vi "BMP180 Pull Raw Measurement.vi"(6 "Sensor Type":enum16{"Temp", "Pressure"}(ring), 8 "error in (no error)":errorcluster, 9 "BMP180 Config":T7={"I2C"={"Slave Address"=64, "Channel"=0}, "Mode"=enum."Ultra Low Power", "Cal Coefs"={"AC1"={"Addr:"=0, "Val:"=0}, "AC2"={"Addr:"=0, "Val:"=0}, "AC3"={"Addr:"=0, "Val:"=0}, "AC4"={"Addr:"=0, "Val:"=0}, "AC5"={"Addr:"=0, "Val:"=0}, "AC6"={"Addr:"=0, "Val:"=0}, "B1"={"Addr:"=0, "Val:"=0}, "B2"={"Addr:"=0, "Val:"=0}, "MB"={"Addr:"=0, "Val:"=0}, "MC"={"Addr:"=0, "Val:"=0}, "MD"={"Addr:"=0, "Val:"=0}}} {"I2C"."Slave Address" format="%.0x"; "Cal Coefs"."MD"."Val:" format="%04x"; "Cal Coefs"."MD"."Addr:" format="%02x"; "Cal Coefs"."MC"."Val:" format="%04x"; "Cal Coefs"."MC"."Addr:" format="%02x"; "Cal Coefs"."MB"."Val:" format="%04x"; "Cal Coefs"."MB"."Addr:" format="%02x"; "Cal Coefs"."B2"."Val:" format="%04x"; "Cal Coefs"."B2"."Addr:" format="%02x"; "Cal Coefs"."B1"."Val:" format="%04x"; "Cal Coefs"."B1"."Addr:" format="%02x"; "Cal Coefs"."AC6"."Val:" format="%04x"; "Cal Coefs"."AC6"."Addr:" format="%02x"; "Cal Coefs"."AC5"."Val:" format="%04x"; "Cal Coefs"."AC5"."Addr:" format="%02x"; "Cal Coefs"."AC4"."Val:" format="%04x"; "Cal Coefs"."AC4"."Addr:" format="%02x"; "Cal Coefs"."AC3"."Val:" format="%04x"; "Cal Coefs"."AC3"."Addr:" format="%02x"; "Cal Coefs"."AC2"."Val:" format="%04x"; "Cal Coefs"."AC2"."Addr:" format="%02x"; "Cal Coefs"."AC1"."Val:" format="%04x"; "Cal Coefs"."AC1"."Addr:" format="%02x"}, 11 "LINX Resource in":T1) -> (0 "error out":errorcluster, 2 "Raw Reading":i32, 3 "LINX Resource":T1)   [LabVIEW 2014]
uses:
  BMP180 Config Options.ctl
  <vilib>/MakerHub/LINX/Private/Type Defs/LINX Ref.ctl
  <vilib>/MakerHub/LINX/Private/Type Defs/Platform.ctl
  <vilib>/MakerHub/LINX/Private/Type Defs/Interface.ctl
  <vilib>/MakerHub/LINX/Private/Device/Type Defs/LINX Device Config.ctl
  <vilib>/MakerHub/LINX/Private/Device/Type Defs/TCP Config.ctl
  <vilib>/MakerHub/LINX/Private/Device/Type Defs/Channels.ctl
  <vilib>/MakerHub/LINX/LMH-LINX.lvlib
  <vilib>/MakerHub/LINX/Private/Device/Device.lvlib
panel:
  out "Data":u8[](array[numeric]) format="%.0x"
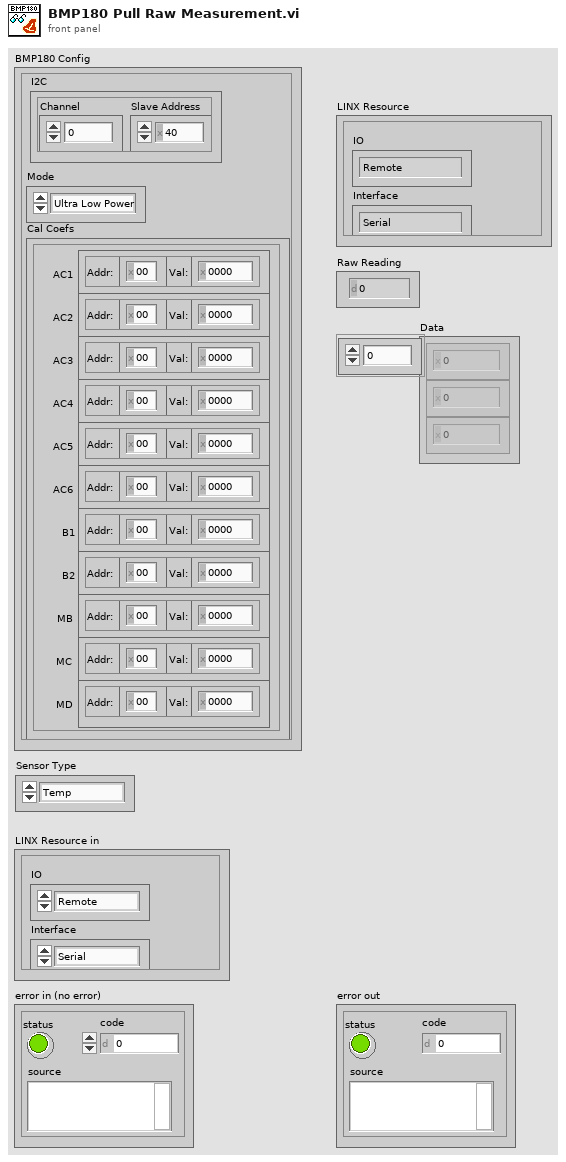
[diagram p1: front panel]
types:
  T1 = typedef "LMH-LINX.lvlib/LINX Ref.ctl" = cluster{"IO":T2, "Interface":T3, "LINX Device Config":T4}
  T2 = typedef "LMH-LINX.lvlib/Platform.ctl" = enum16{"Remote", "Local"}
  T3 = typedef "LMH-LINX.lvlib/Interface.ctl" = enum16{"Serial", "TCP"}
  T4 = typedef "LMH-LINX.lvlib/Device.lvlib/LINX Device Config.ctl" = cluster{"Interface":T3, "COM Port":refnum<visa-resource-name>, "TCP Configuration":T5, "Device Family":u8, "Device ID":u8, "Device Name":string, "TCP Ref":refnum<k5>, "Channels":T6}
  T5 = typedef "LMH-LINX.lvlib/Device.lvlib/TCP Config.ctl" = cluster{"IP Address":string, "Port":u16}
  T6 = typedef "LMH-LINX.lvlib/Channels.ctl" = cluster{"DI":u8[], "DO":u8[], "AI":u8[], "AO":u8[], "PWM":u8[], "QE":u8[], "UART":u8[], "I2C 2":u8[], "SPI":u8[], "CAN":u8[], "Servo":u8[], "AI Ref (V)":dbl, "AI Resolution (Bits)":u8, "AO Ref (V)":dbl, "AO Resolution (Bits)":u8}
  T7 = typedef "BMP180 Config Options.ctl" = cluster{"I2C":cluster{"Slave Address":u8, "Channel":u8}, "Mode":enum8{"Ultra Low Power", "Standard", "High Resolution", "Ultra High Resolution"}, "Cal Coefs":cluster{"AC1":cluster{"Addr:":u8, "Val:":u16}, "AC2":cluster{"Addr:":u8, "Val:":u16}, "AC3":cluster{"Addr:":u8, "Val:":u16}, "AC4":cluster{"Addr:":u8, "Val:":u16}, "AC5":cluster{"Addr:":u8, "Val:":u16}, "AC6":cluster{"Addr:":u8, "Val:":u16}, "B1":cluster{"Addr:":u8, "Val:":u16}, "B2":cluster{"Addr:":u8, "Val:":u16}, "MB":cluster{"Addr:":u8, "Val:":u16}, "MC":cluster{"Addr:":u8, "Val:":u16}, "MD":cluster{"Addr:":u8, "Val:":u16}}}
  T8 = enum8{"Ultra Low Power", "Standard", "High Resolution", "Ultra High Resolution"}
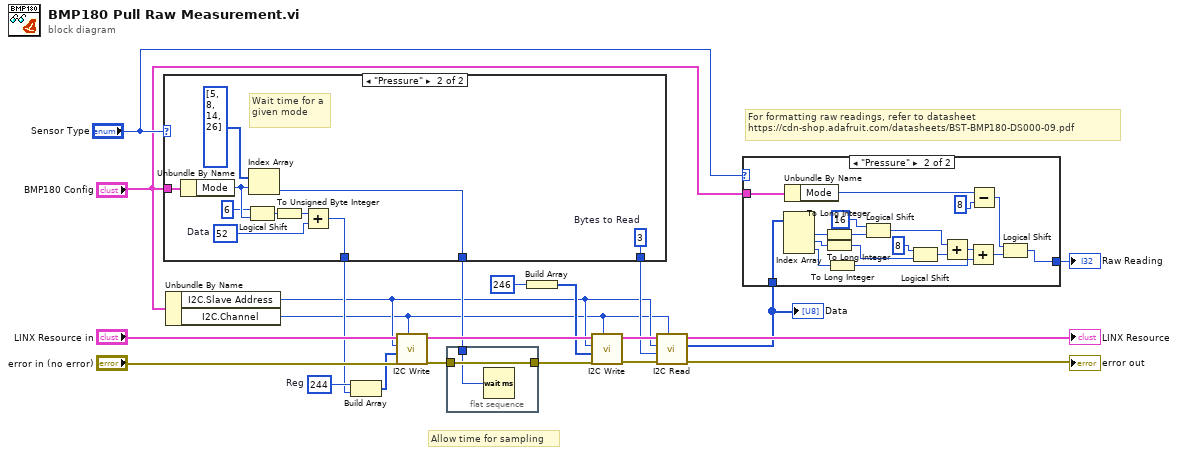
[diagram p0: block diagram]
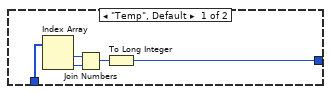
[diagram p2: hidden frame]
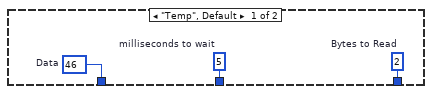
[diagram p3: hidden frame]
diagram:
  w12 = u8 244  # Reg
  # "For formatting raw readings, refer to datasheet\nhttps://cdn-shop.adafruit.com/datasheets/BST-BMP180-DS000-09.pdf"
  # "Allow time for sampling"
  n1 = case shown="\"Pressure\"" "Sensor Type" {
    tunnel: [w25 w33] -> w13
    tunnel: "BMP180 Config" -> [_ w35]
    tunnel: [w24 w27] -> w10
    tunnel: [w23 w26] -> w9
    frame "Temp", Default {
      w23 = u8 2  # Bytes to Read
      w24 = u8 46  # Data
      w25 = u32 5  # milliseconds to wait
    }
    frame "Pressure" {
      w26 = u8 3  # Bytes to Read
      w29 = u8 52  # Data
      # "Wait time for a given mode"
      n2 = Unbundle By Name(w35) -> ("Mode"=w32:T8)
      n3 = Logical Shift(y=i16 6, x=w32) -> (x << y=w30:u32)
      n4 = Index Array(array=u32[] [5, 8, 14, 26], index=w32) -> (element=w33:u32)
      n5 = To Unsigned Byte Integer(number=w30) -> (unsigned 8bit integer=w28:u8)
      n6 = Add(x=w28, y=w29) -> (x+y=w27:u8)
    }
  }
  n7 = Unbundle By Name("BMP180 Config") -> ("I2C.Slave Address"=w2:u8, "I2C.Channel"=w1:u8)
  n8 = Build Array(w12, w10) -> (w11:u8[])
  n9 = call <vilib>:"I2C Write.vi"("I2C Channel"=w1, "Error In"="error in (no error)", "Data"=w11, "I2C Slave Address (0)"=w2, "LINX Resource"="LINX Resource in") -> ("Error Out"=w18:errorcluster, "LINX Resource"=w19:T1)  [unwired: 5 in]
  n10 = flat-sequence {
    tunnel: [w37] -> w20
    tunnel: w18 -> [w37]
    tunnel: w13 -> [w36]
    frame #0 {
      n11 = Wait (ms)(milliseconds to wait=w36) -> ()  [unwired: 1 out]
    }
  }
  n12 = Build Array(u8 246 ("I2C Slave Address 2")) -> (w5:u8[])
  n13 = call <vilib>:"I2C Write.vi"("I2C Channel"=w1, "Error In"=w20, "Data"=w5, "I2C Slave Address (0)"=w2, "LINX Resource"=w19) -> ("Error Out"=w21:errorcluster, "LINX Resource"=w22:T1)  [unwired: 5 in]
  n14 = call <vilib>:"I2C Read.vi"("I2C Channel"=w1, "Error In"=w21, "Bytes To Read"=w9, "I2C Slave Address (0)"=w2, "LINX Resource"=w22) -> ("Error Out"=→"error out":errorcluster, "Data"=w7:u8[], "LINX Resource"=→"LINX Resource":T1)  [unwired: 4 in]
  "Data" <- w7
  n15 = case shown="\"Pressure\"" "Sensor Type" {
    tunnel: w7 -> [w39 w60]
    tunnel: "BMP180 Config" -> [_ w59]
    tunnel: [w38 w43] -> w4
    frame "Temp", Default {
      n16 = Index Array(array=w39) -> (element #1=w42:u8, element #2=w41:u8)  [unwired: 2 in]
      n17 = Join Numbers(hi=w42, lo=w41) -> ((hi.lo)=w40:u16)
      n18 = To Long Integer(number=w40) -> (32bit integer=w38:i32)
    }
    frame "Pressure" {
      n19 = Index Array(array=w60) -> (element #1=w58:u8, element #2=w52:u8, element #3=w50:u8)  [unwired: 3 in]
      n20 = Unbundle By Name(w59) -> ("Mode"=w46:T8)
      n21 = To Long Integer(number=w58) -> (32bit integer=w57:i32)
      n22 = To Long Integer(number=w52) -> (32bit integer=w51:i32)
      n23 = To Long Integer(number=w50) -> (32bit integer=w49:i32)
      n24 = Logical Shift(y=i16 16, x=w57) -> (x << y=w54:i32)
      n25 = Logical Shift(y=i16 8, x=w51) -> (x << y=w55:i32)
      n26 = Add(x=w54, y=w55) -> (x+y=w48:i32)
      n27 = Add(x=w48, y=w49) -> (x+y=w47:i32)
      n28 = Subtract(x=w46, y=i16 8) -> (x-y=w44:i16)
      n29 = Logical Shift(y=w44, x=w47) -> (x << y=w43:i32)
    }
  }
  "Raw Reading" <- w4
